vi "GEOM_GetWCSFile.vi"(10 "wcs":string) -> (2 "file out":path)   [LabVIEW 2016]
uses:
  GEOM_VAR_action.ctl
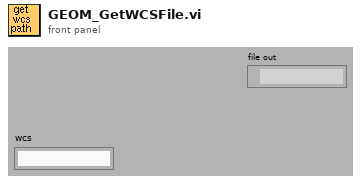
[diagram p1: front panel]
types:
  T1 = typedef "GEOM_VAR_action.ctl" = enum16{"read", "write"}
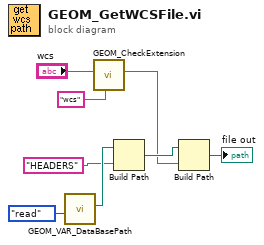
[diagram p0: block diagram]
diagram:
  n1 = call "GEOM_VAR_DataBasePath.vi"("Action"=GEOM_VAR_action."read") -> ("GEOM_coordsref out"=w7:path)  [unwired: 1 in, 9 out]
  n2 = call "GEOM_CheckExtension.vi"("extension to look"="wcs", "name in"="wcs") -> ("name out"=w2:string)  [unwired: 8 out]
  n3 = Build Path(base path=w7, name or relative path="HEADERS") -> (appended path=w3:path)
  n4 = Build Path(base path=w3, name or relative path=w2) -> (appended path=→"file out":path)
